vi "Clear Route.vi"(7 "Clear Polygon?":bool=TRUE, 8 "Error In":errorcluster, 11 "Route Index":i32) -> (0 "error out":errorcluster)   [LabVIEW 2014]
uses:
  C:/Robotic Systems/Products/AgFalcon/Software/Ground Station/Data/Mapping DLL/GMap.NET.WindowsForms.dll
  Data/Mapping DLL/GMap.NET.WindowsForms.dll
  Reference/SubVI/GMap DLL Refernce.vi
  Reference/SubVI/Main Map Control Refernce.vi
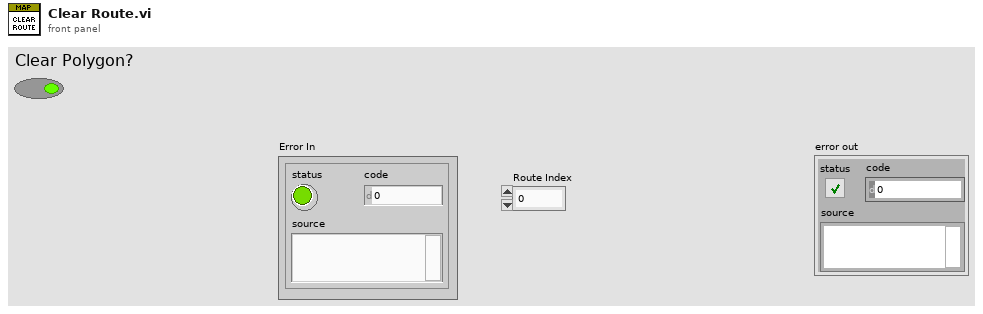
[diagram p1: front panel]
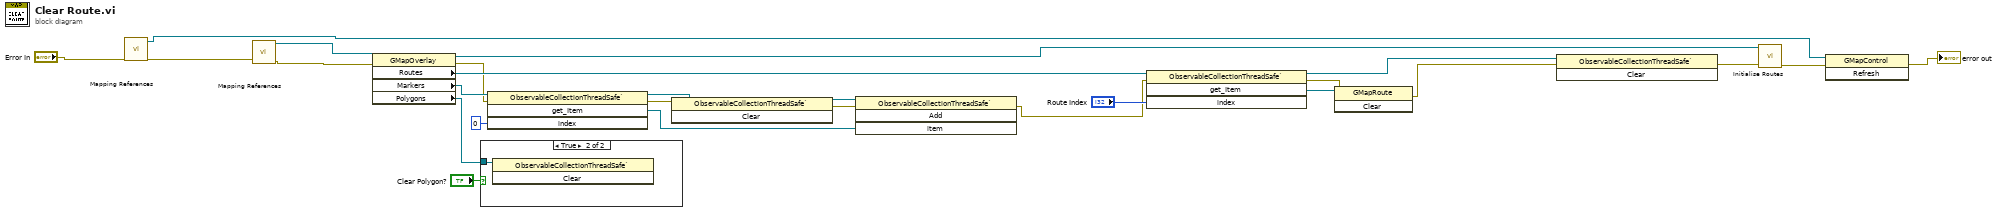
[diagram p0: block diagram]
diagram:
  n1 = call-poly "Mapping References.vi"("Error In"="Error In") -> ("Error Out"=w19:errorcluster, "GMap DLL Reference"=w17:refnum<k24>)  [unwired: 9 in]
  n2 = call-poly "Mapping References.vi"("Error In"=w19) -> ("Error Out"=w24:errorcluster, "Main Map Reference"=w20:refnum<k24>)  [unwired: 9 in]
  n3 = property class="GMapOverlay"(reference=w20, error in=w24) -> (reference out=w13:refnum<k24>, error out=w10:errorcluster, "Routes"=w25:refnum<k24>, "Markers"=w11:refnum<k24>, "Polygons"=w2:refnum<k24>)
  n4 = case shown="True" "Clear Polygon?" {
    tunnel: w2 -> [_ w27]
    frame False {
    }
    frame True {
      n5 = invoke class="ObservableCollectionThreadSafe`" method="Clear"(reference=w27) -> ()  [unwired: 2 in, 3 out]
    }
  }
  n6 = invoke class="ObservableCollectionThreadSafe`" method="get_Item"(reference=w11, error in=w10, "index"=0) -> (reference out=w8:refnum<k24>, error out=w7:errorcluster, "get_Item"=w4:refnum<k24>)  [unwired: 1 in, 1 out]
  n7 = invoke class="ObservableCollectionThreadSafe`" method="Clear"(reference=w8, error in=w7) -> (reference out=w6:refnum<k24>, error out=w5:errorcluster)  [unwired: 1 in, 1 out]
  n8 = invoke class="ObservableCollectionThreadSafe`" method="Add"(reference=w6, error in=w5, "item"=w4) -> (error out=w3:errorcluster)  [unwired: 1 in, 3 out]
  n9 = invoke class="ObservableCollectionThreadSafe`" method="get_Item"(reference=w25, error in=w3, "index"="Route Index") -> (reference out=w14:refnum<k24>, error out=w22:errorcluster, "get_Item"=w23:refnum<k24>)  [unwired: 1 in, 1 out]
  n10 = invoke class="GMapRoute" method="Clear"(reference=w23, error in=w22) -> (error out=w12:errorcluster)  [unwired: 1 in, 2 out]
  n11 = invoke class="ObservableCollectionThreadSafe`" method="Clear"(reference=w14, error in=w12) -> (error out=w15:errorcluster)  [unwired: 1 in, 2 out]
  n12 = call "Initialise Routes.vi"("error in (no error)"=w15, "Main Overlay"=w13) -> ("error out"=w16:errorcluster)  [unwired: 9 in]
  n13 = invoke class="GMapControl" method="Refresh"(reference=w17, error in=w16) -> (error out=→"error out":errorcluster)  [unwired: 1 in, 2 out]
